vi "CalculateTargetSpeed.vi"(8 "Target Edge Pos. (mm)":dbl, 9 "Shooting Pos. (mm)":dbl, 10 "Target Radius (mm)":dbl, 11 "Shot Spacing (mm)":dbl) -> (1 "Numeric Control 2":dbl, 2 "Numeric Control 3":dbl, 3 "Numeric Control":dbl)   [LabVIEW 2014, in "ShootingStar.lvlib"]
uses:
  ShootingStar.lvlib
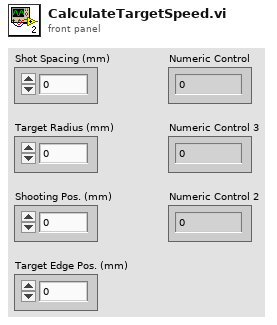
[diagram p1: front panel]
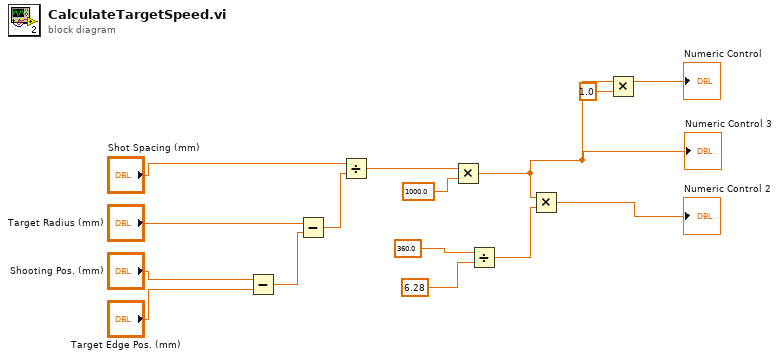
[diagram p0: block diagram]
diagram:
  n1 = Subtract(x="Shooting Pos. (mm)", y="Target Edge Pos. (mm)") -> (x-y=w1:dbl)
  n2 = Subtract(x="Target Radius (mm)", y=w1) -> (x-y=w2:dbl)
  n3 = Divide(x="Shot Spacing (mm)", y=w2) -> (x/y=w3:dbl)
  n4 = Multiply(x=w3, y=1000.0) -> (x*y=w12:dbl)
  "Numeric Control 3" <- w12
  n5 = Divide(x=360.0, y=6.28 ("x")) -> (x/y=w7:dbl)
  n6 = Multiply(x=w12, y=w7) -> (x*y=→"Numeric Control 2":dbl)
  n7 = Multiply(x=w12, y=1.0) -> (x*y=→"Numeric Control":dbl)
